vi "Update FPGA.vi"(8 "error in":errorcluster, 9 "Samples per Cycle":u16, 10 "RepRate":u16, 11 "gCRDS":refnum<class "gCRD.lvclass">) -> (0 "error out":errorcluster, 3 "gCRDS":refnum<class "gCRD.lvclass">)   [LabVIEW 2017, in "gCRDS.lvlib" / "Change Laser Rep Rate CMD.lvclass"]
uses:
  Change Laser Rep Rate CMD.lvclass
  gCRD.lvclass
  gCRD.lvclass/gCRD.ctl
  Accessors/Read hFPGA.vi
  <vilib>/Utility/error.llb/Error Cluster From Error Code.vi
  <vilib>/rvi/errors/niLvFpgaAdjustHostInterfaceError.vi
  <vilib>/MSR Consulting, LLC/General Reuse/Session APIs/_Session Fwk/Session - Root.lvclass
  <vilib>/rvi/interface/nirviReadWriteControl/nirviReadWriteControl.xnode
  FPGA Ref.ctl
  FPGA Bitfiles/server.lvbitx
  Session/Raw FPGA/FPGA Session.lvclass
  NiFpgaLv.dll
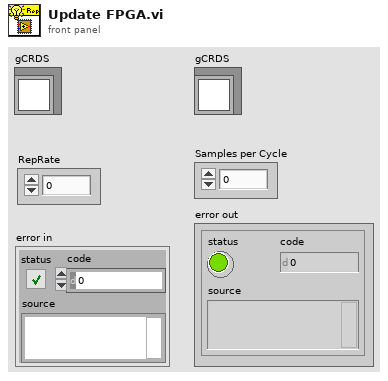
[diagram p1: front panel]
types:
  T1 = typedef "Session - Root.lvclass/Session Handle.ctl" = refnum<data-value>
  T2 = typedef "FPGA Ref.ctl" = refnum<k20>
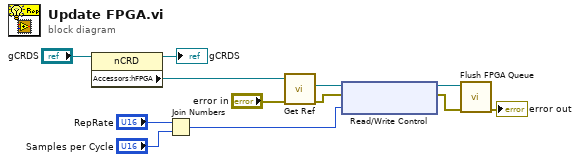
[diagram p0: block diagram]
diagram:
  n1 = property class="nCRD"(reference="gCRDS") -> (reference out=→"gCRDS":refnum<class "gCRD.lvclass">, "Accessors:hFPGA"=w8:T1)  [unwired: 1 in, 1 out]
  n2 = Join Numbers(hi="RepRate", lo="Samples per Cycle") -> ((hi.lo)=w6:u32)
  n3 = call "Get Ref.vi"("error in"="error in", "Hanlde Out"=w8) -> ("error out"=w12:errorcluster, "FPGA Ref"=w11:T2)  [unwired: 7 in, 1 out]
  n4 = xnode "Read/Write Control"("FPGA VI Reference In"=w11, "error in"=w12, "CRDSampData"=w6) -> ("FPGA VI Reference Out"=w3:T2, "error out"=w2:errorcluster)
  n5 = call "Flush FPGA Queue.vi"("error in"=w2, "Refnum in"=w3) -> ("error out"=→"error out":errorcluster)  [unwired: 9 in]
